vi "Query.vi"(8 "error in (no error)":errorcluster, 10 "Cmd":string, 11 "NRT8000 in":refnum<class "NRT8000.lvclass">) -> (0 "error out":errorcluster, 2 "Rsp":string, 3 "NRT8000 out":refnum<class "NRT8000.lvclass">)   [LabVIEW 2018, in "NRT8000.lvlib" / "NRT8000.lvclass"]
uses:
  NRT8000.lvclass
  PPLs/Optical Spectrum Analyzer/Parent/OSA.lvlibp/Optical Spectrum Analyzer.lvclass
  C:/Projects/LabVIEW/PPLs/Optical Spectrum Analyzer/Parent/OSA.lvlibp/Optical Spectrum Analyzer.lvclass
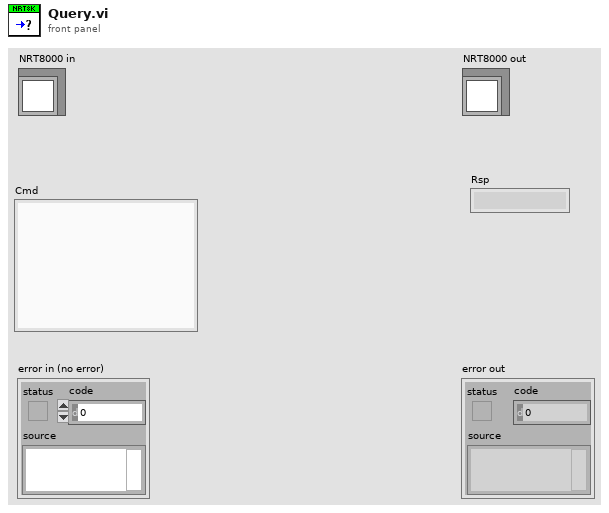
[diagram p1: front panel]
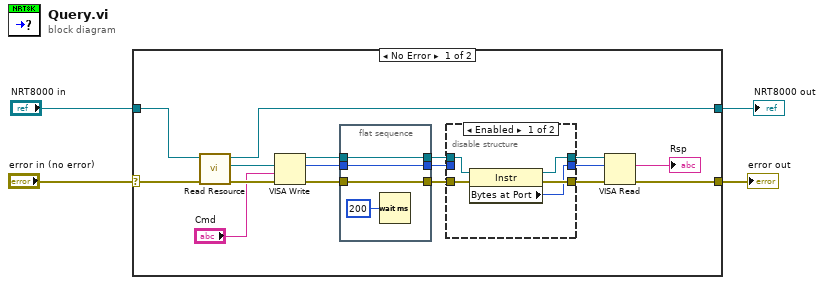
[diagram p0: block diagram]
diagram:
  n1 = case shown="No Error" "error in (no error)" {
    selector: "error in (no error)" -> [w21 w35]
    tunnel: [w12 w35] -> w3
    tunnel: [w17 w34] -> w1
    tunnel: "NRT8000 in" -> [w20 w34]
    frame No Error {
      n2 = call "Read Resource.vi"("error in (no error)"=w21, "Optical Spectrum Analyzer in"=w20) -> ("error out"=w19:errorcluster, "Resource"=w18:refnum<visa-resource-name>, "Optical Spectrum Analyzer out"=w17:refnum<class "NRT8000.lvclass">)  [unwired: 7 in]
      n3 = VISA Write(VISA resource name=w18, write buffer="Cmd", error in (no error)=w19) -> (VISA resource name out=w10:refnum<visa-resource-name>, return count=w6:u32, error out=w8:errorcluster)
      n4 = flat-sequence {
        tunnel: w10 -> [w25]
        tunnel: [w25] -> w9
        tunnel: w8 -> [w24]
        tunnel: [w24] -> w7
        tunnel: w6 -> [w22]
        tunnel: [w22] -> w5
        frame #0 {
          n5 = Wait (ms)(milliseconds to wait=u32 200) -> ()  [unwired: 1 out]
        }
      }
      n6 = disable-structure shown="Enabled" {
        disable-tunnel: [w30 w31] -> w15
        disable-tunnel: [w29 w33] -> w14
        disable-tunnel: [w28 w32] -> w13
        disable-tunnel: w9 -> [w27 w33]
        disable-tunnel: w7 -> [w26 w31]
        disable-tunnel: w5 -> [_ w32]
        frame Enabled {
          n7 = property class="Instr"(reference=w27, error in=w26) -> (reference out=w29:refnum<visa-resource-name>, error out=w30:errorcluster, "Bytes at Port"=w28:u32)
        }
        frame Disabled {
        }
      }
      n8 = VISA Read(VISA resource name=w14, byte count=w13, error in (no error)=w15) -> (read buffer=→"Rsp":string, error out=w12:errorcluster)  [unwired: 2 out]
    }
    frame Error {
    }
  }
  "error out" <- w3
  "NRT8000 out" <- w1
